vi "DiffX.vi"(2 "Array in":dbl[][](array[numeric]), 3 "DiffX":bool caption="Scan") -> (0 "Array out":dbl[][](array[numeric]))   [LabVIEW 2018]
uses:
  <vilib>/Analysis/NI_AALPro.lvlib
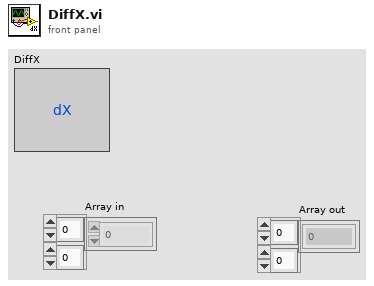
[diagram p1: front panel]
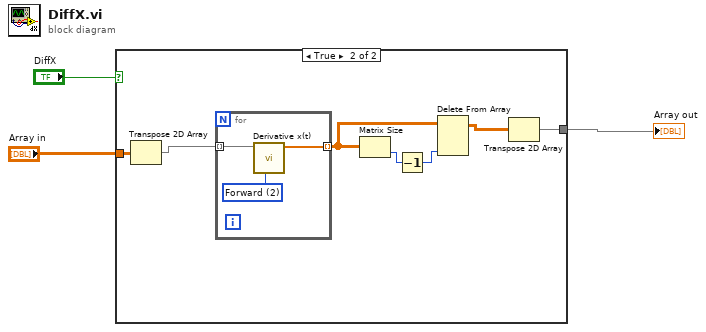
[diagram p0: block diagram]
diagram:
  n1 = case shown="True" "DiffX" {
    tunnel: "Array in" -> [w4 w8]
    tunnel: [w4 w5] -> w1
    frame False {
    }
    frame True {
      n2 = Transpose 2D Array(2D array=w8) -> (transposed array=w7:dbl[][])
      n3 = for {
        tunnel: w7 -> [w14] mode=indexing
        tunnel: [w12] -> w11 mode=indexing
        w13 = u16 2 items=["2nd Order Central", "4th Order Central", "Forward", "Backward"] ("method")
        n4 = call <vilib>:"Derivative x(t).vi"("method"=w13, "X"=w14) -> ("dX/dt"=w12:dbl[])  [unwired: 8 in, 1 out]
      }
      n5 = Matrix Size(0:w11) -> (2:w9:i32)  [unwired: 1 out]
      n6 = Decrement(x=w9) -> (x-1=w10:i32)
      n7 = Delete From Array(array=w11, index (col)=w10) -> (array with subset deleted=w6:dbl[][])  [unwired: 2 in, 1 out]
      n8 = Transpose 2D Array(2D array=w6) -> (transposed array=w5:dbl[][])
    }
  }
  "Array out" <- w1
